vi "Update Ball Position.vi"(8 "Cluster width":i32=200, 9 "Ball Nr":i32, 10 "Ball Refs":refnum<vi>[](array[refnum]), 11 "Position In":i32) -> (3 "Position out":i32)   [LabVIEW 2014, in "Endigit.lvlib"]
uses:
  Endigit.lvlib
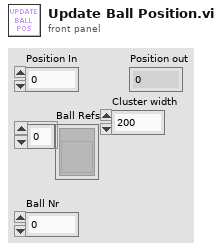
[diagram p1: front panel]
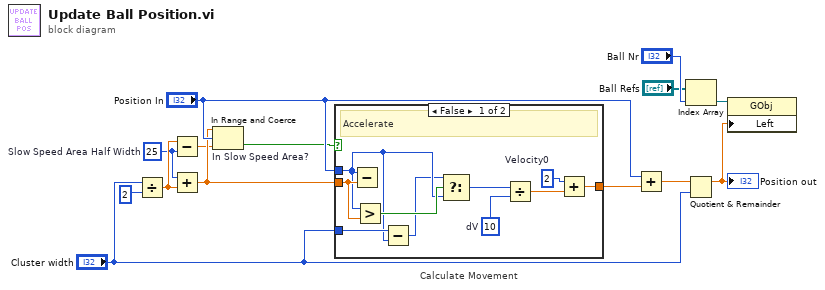
[diagram p0: block diagram]
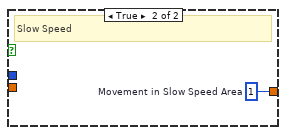
[diagram p2: hidden frame]
diagram:
  w3 = 25  # Slow Speed Area Half Width
  n1 = Divide(x="Cluster width", y=2) -> (x/y=w5:dbl)
  n2 = Subtract(x=w5, y=w3) -> (x-y=w4:dbl)
  n3 = Add(x=w3, y=w5) -> (x+y=w7:dbl)
  n4 = In Range and Coerce "In Slow Speed Area?"(upper limit=w7, x="Position In", lower limit=w4) -> (In Range?=w10:bool)  [unwired: 1 out]
  n5 = case "Calculate Movement" shown="False" w10 {
    tunnel: [w23 w25] -> w1
    tunnel: "Position In" -> [w16 _]
    tunnel: w7 -> [w19 _]
    tunnel: "Cluster width" -> [w17 _]
    frame False {
      w20 = 10  # dV
      w24 = 2  # Velocity0
      # "Accelerate"
      n6 = Subtract(x=w16, y=w19) -> ()  [unwired: 1 out]
      n7 = Greater?(x=w16, y=w19) -> (0:w22:bool)
      n8 = Subtract(x=w17, y=w16) -> (x-y=w15:i32)
      n9 = Select(t=w15, s=w22, f=w16) -> (s? t:f=w21:i32)
      n10 = Divide(x=w21, y=w20) -> (x/y=w18:dbl)
      n11 = Add(x=w24, y=w18) -> (x+y=w23:dbl)
    }
    frame True {
      w25 = 1  # Movement in Slow Speed Area
      # "Slow Speed"
    }
  }
  n12 = Add(x="Position In", y=w1) -> (x+y=w9:dbl)
  n13 = Index Array(array="Ball Refs", index="Ball Nr") -> (element=w12:refnum<vi>)
  n14 = Quotient & Remainder(x=w9, y="Cluster width") -> (x-y*floor(x/y)=w8:dbl)  [unwired: 1 out]
  "Position out" <- w8
  n15 = property class="GObj"(reference=w12, "Left"=w8) -> ()  [unwired: 1 in, 2 out]
